vi "COMMOut.vi"(0 "Numeric":i16, 1 "VISA resource name":refnum<visa-resource-name>) -> ()   [LabVIEW 2025]
panel:
  # "Data Aquisition Package - LabView and the NAIT Micro11 Board"
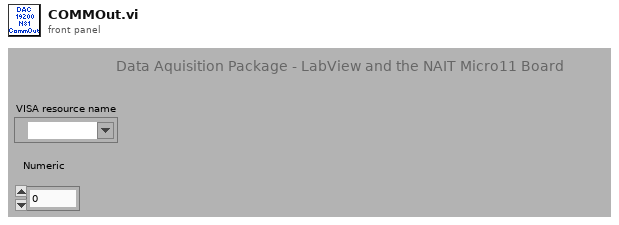
[diagram p1: front panel]
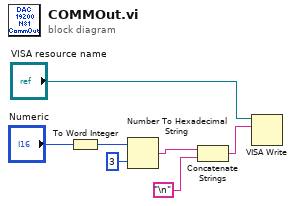
[diagram p0: block diagram]
diagram:
  n1 = To Word Integer(number="Numeric") -> (16bit integer=w5:i16)
  n2 = Number To Hexadecimal String(1:i16 3 ("width (-)"), 2:w5) -> (0:w3:string)
  n3 = Concatenate Strings(w3, "\n") -> (w1:string)
  n4 = VISA Write(VISA resource name="VISA resource name", write buffer=w1) -> ()  [unwired: 1 in, 3 out]
